vi "Graphics-Autoscale.vi"(8 "error in (no error)":errorcluster, 9 "Resolution":dbl, 10 "Value":cluster{"X":dbl[], "Y":dbl[]}[](array[cluster]), 11 "XYGraph in":refnum<vi>) -> (0 "error out":errorcluster)   [LabVIEW 2020]
panel:
  out "XYGraph out":refnum<vi>
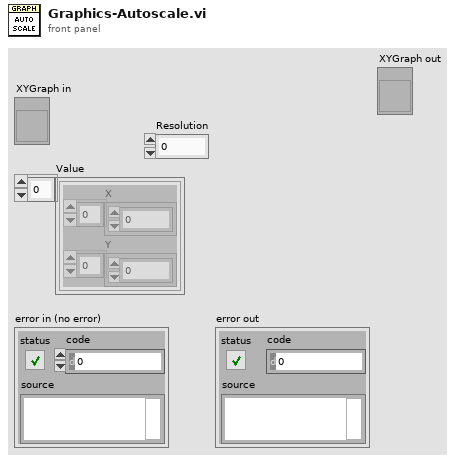
[diagram p1: front panel]
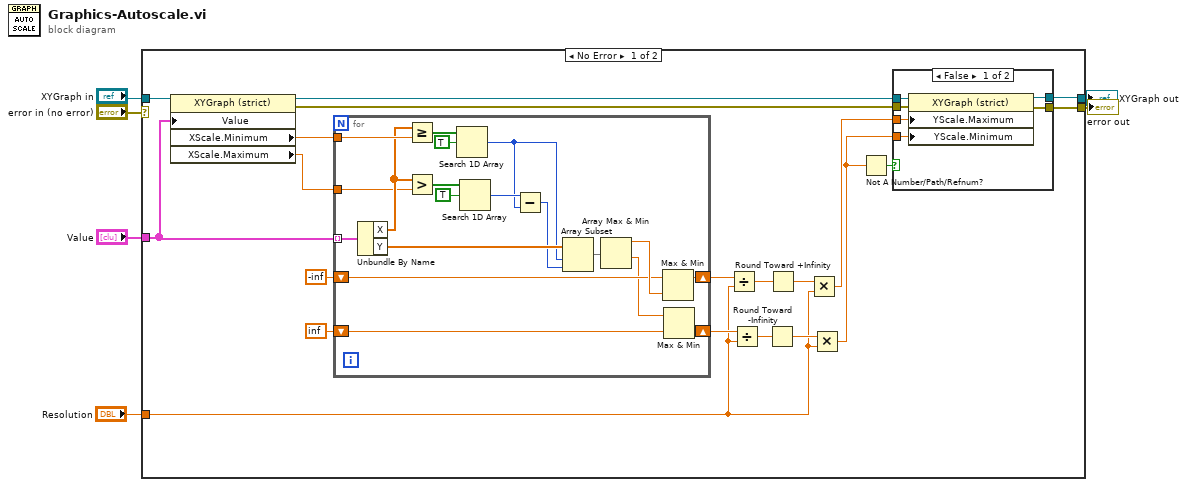
[diagram p0: block diagram]
diagram:
  n1 = case shown="No Error" "error in (no error)" {
    selector: "error in (no error)" -> [_ w55]
    tunnel: "XYGraph in" -> [w26 w54]
    tunnel: "Value" -> [w25 _]
    tunnel: [w19 w55] -> w5
    tunnel: [w20 w54] -> w2
    tunnel: "Resolution" -> [w10 _]
    frame No Error {
      n2 = property class="XYGraph (strict)"(reference=w26, "Value"=w25) -> (reference out=w22:refnum<vi>, error out=w21:errorcluster, "XScale.Minimum"=w24:dbl, "XScale.Maximum"=w23:dbl)  [unwired: 1 in]
      n3 = for {
        tunnel: w25 -> [w53] mode=indexing
        tunnel: w24 -> [w52]
        tunnel: w23 -> [w48]
        shift-right: [w40] -> w16
        shift-left: -inf -> [w36]
        shift-right: [w39] -> w13
        shift-left: inf -> [w38]
        n4 = Unbundle By Name(w53) -> ("X"=w49:dbl[], "Y"=w44:dbl[])
        n5 = Greater Or Equal?(x=w49, y=w52) -> (x >= y?=w51:bool[])
        n6 = Greater?(x=w49, y=w48) -> (0:w47:bool[])
        n7 = Search 1D Array(1D array=w51, element=TRUE) -> (index of element=w43:i32)  [unwired: 1 in]
        n8 = Search 1D Array(1D array=w47, element=TRUE) -> (index of element=w45:i32)  [unwired: 1 in]
        n9 = Subtract(x=w45, y=w43) -> (x-y=w42:i32)
        n10 = Array Subset(array=w44, index=w43, length=w42) -> (w41:dbl[])
        n11 = Array Max & Min(array=w41) -> (max value=w37:dbl, min value=w35:dbl)  [unwired: 2 out]
        n12 = Max & Min(x=w36, y=w37) -> (max(x,y)=w40:dbl)  [unwired: 1 out]
        n13 = Max & Min(x=w35, y=w38) -> (min(x,y)=w39:dbl)  [unwired: 1 out]
      }
      n14 = Divide(x=w16, y=w10) -> (x/y=w15:dbl)
      n15 = Divide(x=w13, y=w10) -> (x/y=w12:dbl)
      n16 = Round Toward -Infinity(1:w12) -> (0:w11:dbl)
      n17 = Round Toward +Infinity(x=w15) -> (ceil(x): smallest int >= x=w14:dbl)
      n18 = Multiply(x=w14, y=w10) -> (x*y=w9:dbl)
      n19 = Multiply(x=w11, y=w10) -> (x*y=w7:dbl)
      n20 = Not A Number/Path/Refnum?(number/path/refnum=w7) -> (NaN/Path/Refnum?=w8:bool)
      n21 = case shown="False" w8 {
        tunnel: w22 -> [w32 w34]
        tunnel: w21 -> [w31 w33]
        tunnel: [w30 w34] -> w20
        tunnel: [w29 w33] -> w19
        tunnel: w9 -> [w28 _]
        tunnel: w7 -> [w27 _]
        frame False {
          n22 = property class="XYGraph (strict)"(reference=w32, error in=w31, "YScale.Maximum"=w28, "YScale.Minimum"=w27) -> (reference out=w30:refnum<vi>, error out=w29:errorcluster)
        }
        frame True {
        }
      }
    }
    frame Error {
    }
  }
  "error out" <- w5
  "XYGraph out" <- w2
